vi "ERR Build Call Chain from Source.vi"(0 "Error Source":string) -> (4 "Call Chain":string[](array[string]))   [LabVIEW 2011]
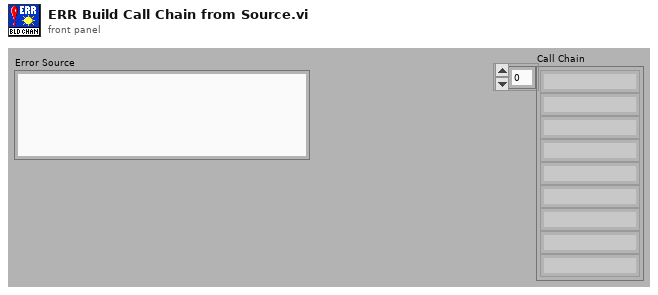
[diagram p1: front panel]
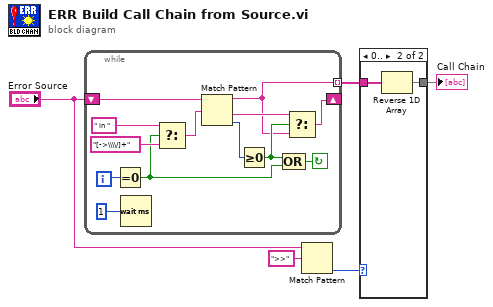
[diagram p0: block diagram]
diagram:
  n1 = while {
    tunnel: [w8] -> w3 mode=indexing
    shift-left: "Error Source" -> [w16]
    shift-right: [w7] -> _
    i -> [w15]
    stop <- w11 continue-if-true
    n2 = Equal To 0?(x=w15) -> (x = 0?=w6:bool)
    n3 = Wait (ms)(milliseconds to wait=u32 1) -> ()  [unwired: 1 out]
    n4 = Select(t=" in " ("regular expression"), s=w6, f="[->\\\\/]+" ("regular expression")) -> (s? t:f=w12:string)
    n5 = Match Pattern(string=w16, regular expression=w12) -> (before substring=w8:string, after substring=w9:string, offset past match=w17:i32)  [unwired: 2 out]
    n6 = Greater Or Equal To 0?(x=w17) -> (x >= 0?=w10:bool)
    n7 = Compound Arithmetic op=OR(w10, w6) -> (w11:bool)
    n8 = Select(t=w9, s=w10, f=w8) -> (s? t:f=w7:string)
  }
  n9 = Match Pattern(string="Error Source", regular expression=">>") -> (offset past match=w4:i32)  [unwired: 4 out]
  n10 = case shown="0.." w4 {
    tunnel: w3 -> [w19 w21]
    tunnel: [w19 w20] -> w2
    frame ..-1 {
    }
    frame 0.. {
      n11 = Reverse 1D Array(array=w21) -> (reversed array=w20:string[])
    }
  }
  "Call Chain" <- w2
